vi "ReportIdentification.vi"(7 "Vehicle Name":string="Q", 8 "Destination":T1={"Subsystem Id"=90, "Node Id"=1, "Component Id"=1}, 9 "Type":u16=10001, 10 "QueryType":u8=2, 11 "Source":T1={"Subsystem Id"=3, "Node Id"=1, "Component Id"=1}) -> (3 "Encoded JAUS Message":string)   [LabVIEW 2009]
uses:
  Support Files/Address.ctl
panel:
  in  "Command Code":string="K\u0000"
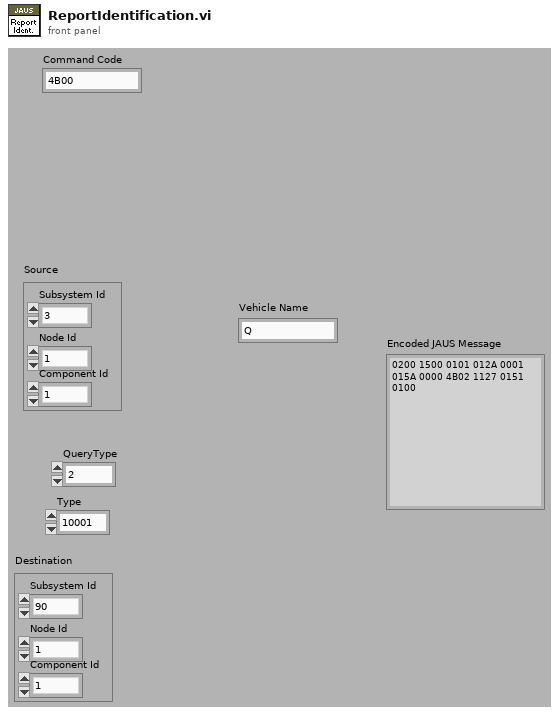
[diagram p1: front panel]
types:
  T1 = typedef "Address.ctl" = cluster{"Subsystem Id":u16, "Node Id":u8, "Component Id":u8}
  T2 = cluster{"unsigned byte array[0]":u8, "unsigned byte array[1]":u8}
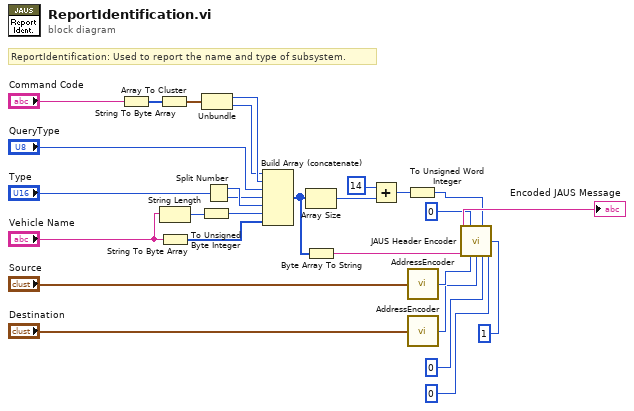
[diagram p0: block diagram]
diagram:
  # "ReportIdentification: Used to report the name and type of subsystem."
  n1 = String To Byte Array(string="Command Code") -> (unsigned byte array=w11:u8[])
  n2 = Array To Cluster(array=w11) -> (cluster=w10:T2)
  n3 = String Length(string="Vehicle Name") -> (length=w16:i32)
  n4 = String To Byte Array(string="Vehicle Name") -> (unsigned byte array=w18:u8[])
  n5 = To Unsigned Byte Integer(number=w16) -> (unsigned 8bit integer=w17:u8)
  n6 = Unbundle(w10) -> ("unsigned byte array[0]"=w9:u8, "unsigned byte array[1]"=w8:u8)
  n7 = Split Number(x="Type") -> (hi(x)=w13:u8, lo(x)=w12:u8)
  n8 = Build Array (concatenate)(w8, w9, "QueryType", w12, w13, w17, w18) -> (w7:u8[])
  n9 = Array Size(array=w7) -> (size(s)=w6:i32)
  n10 = Byte Array To String(unsigned byte array=w7) -> (string=w20:string)
  n11 = Add(x=14 ("Data Size (8-23)"), y=w6) -> (x+y=w4:i32)
  n12 = To Unsigned Word Integer(number=w4) -> (unsigned 16bit integer=w1:u16)
  n13 = call "AddressEncoder.vi"("Address Cluster"="Source") -> ("Address"=w27:u32)
  n14 = call "AddressEncoder.vi"("Address Cluster"="Destination") -> ("Address"=w26:u32)
  n15 = call "JAUS Header Encoder.vi"("Message Type (0-5)"=u8 0, "Data Size (8-23)"=w1, "Priority(40-41)"=u8 1, "Payload"=w20, "Source ID (80-95)"=w27, "Destination ID (48-79)"=w26, "Data Flags (46-47)"=u8 0, "Ack/Nak (44-45)"=u8 0) -> ("Encoded JAUS Message"=→"Encoded JAUS Message":string)  [unwired: 7 in]
